vi "ResetRainEvent.vi"(11 "RainAccumulation":dbl) -> (2 "Elapsed Time (s)":dbl, 3 "Time has Elapsed":bool)   [LabVIEW 2018]
doc: "We are now resetting the \"rain accumulation\" count from the Disdrometer\n15 minutes after a rain event. \nCheck rain accumulation and compare to the previous measurement. If the value has changed, reset the timer.\n\nIf 15 minutes (900 seconds) have elapsed without a change in the measured value, reset the disdrometer accumulation value."
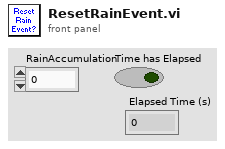
[diagram p1: front panel]
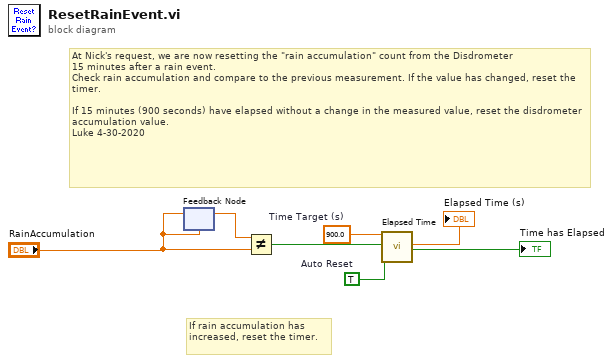
[diagram p0: block diagram]
diagram:
  w6 = TRUE  # Auto Reset
  w4 = 900.0  # Time Target (s)
  # "At Nick's request, we are now resetting the \"rain accumulation\" count from the Disdrometer\n15 minutes after a rain event. \nCheck rain accumulation and compare to the previous measurement. If the value has changed, reset the timer.\n\nIf 15 minutes (900 seconds) have elapsed without a change in the measured value, reset the disdrometer accumulation value.\nLuke 4-30-2020"
  # "If rain accumulation has increased, reset the timer."
  n1 = feedback #1("RainAccumulation") -> (w2:dbl)
  n2 = feedback-in #1("RainAccumulation") -> ()
  n3 = Not Equal?(x=w2, y="RainAccumulation") -> (x != y?=w5:bool)
  n4 = call "Elapsed Time"("Time Target (s)"=w4, "Reset"=w5, "Auto Reset"=w6) -> ("Elapsed Time (s)"=→"Elapsed Time (s)":dbl, "Time has Elapsed"=→"Time has Elapsed":bool)  [unwired: 9 in, 6 out]
